vi "Read Status.vi"(6 "Selector":T1, 8 "error in":errorcluster, 11 "PIOD in":refnum<class "PIOD.lvclass">) -> (0 "error out":errorcluster, 3 "PIOD out":refnum<class "PIOD.lvclass">)   [LabVIEW 2018, in "PIOD.lvlib" / "PIOD.lvclass"]
uses:
  PIOD.lvclass
  PPLs/PLC/Parent/PLC.lvlibp/Custom Controls/Selector.ctl
  PPLs/PLC/Parent/PLC.lvlibp/PLC.lvclass
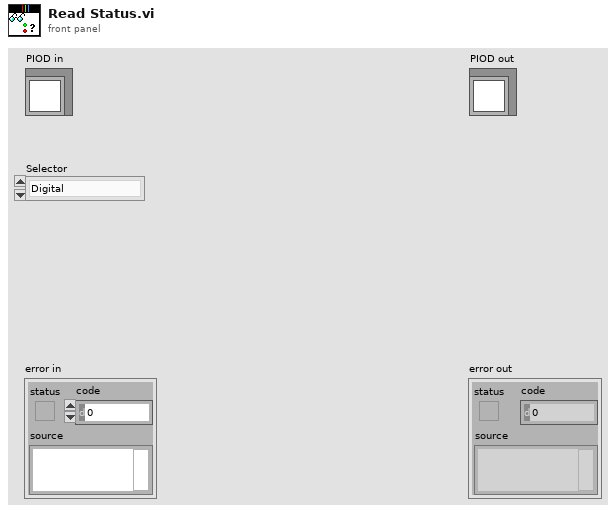
[diagram p1: front panel]
types:
  T1 = typedef "PLC.lvlibp/PLC.lvclass/Selector.ctl" = enum16{"Digital", "Analog"}
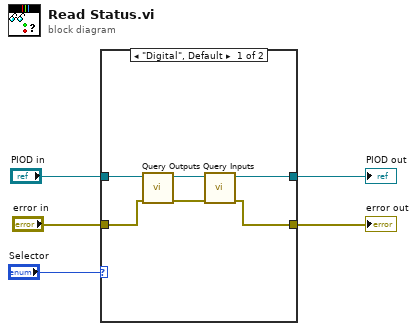
[diagram p0: block diagram]
diagram:
  n1 = case shown="\"Digital\", Default" "Selector" {
    tunnel: "PIOD in" -> [w11 w13]
    tunnel: "error in" -> [w10 w12]
    tunnel: [w7 w13] -> w2
    tunnel: [w6 w12] -> w1
    frame "Digital", Default {
      n2 = call "Query Outputs.vi"("error in"=w10, "PIOD in"=w11) -> ("error out"=w8:errorcluster, "PIOD out"=w9:refnum<class "PIOD.lvclass">)  [unwired: 8 in]
      n3 = call "Query Inputs.vi"("error in"=w8, "PIOD in"=w9) -> ("error out"=w6:errorcluster, "PIOD out"=w7:refnum<class "PIOD.lvclass">)  [unwired: 8 in]
    }
    frame "Analog" {
    }
  }
  "error out" <- w1
  "PIOD out" <- w2
